vi "Test--wink.vi"() -> ()   [LabVIEW 2024, in "Flexi-Flow Modbus TCP API.lvlib"]
uses:
  Flexi-Flow Modbus TCP API.lvlib
  ca-ec-test-stand/Dependencies/gmodbustcp-main/Sources/Lvlib/ModBusVIEWoTCP.lvlib
panel:
  out "Word":i16
  out "Information out":T1 {"Unit identifier" max=247; "exceptionCode" max=247}
  in  "Word address":u16 format="%x"
  in  "Word (0)":i16
  in  "Network":T2={"server address"="192.168.100.10", "remote port (502)"=502}
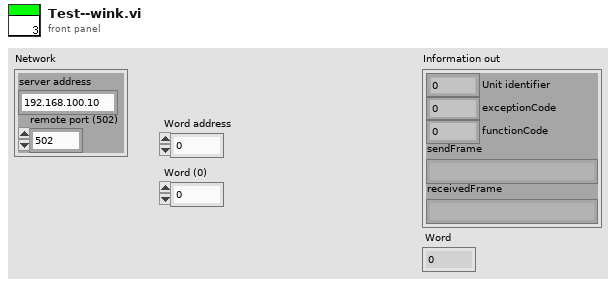
[diagram p1: front panel]
types:
  T1 = cluster{"Unit identifier":u8, "exceptionCode":u8, "functionCode":u8, "sendFrame":string, "receivedFrame":string}
  T2 = cluster{"server address":string, "remote port (502)":u16}
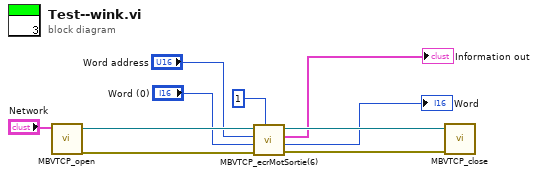
[diagram p0: block diagram]
diagram:
  n1 = call "MBVTCP_open.vi"("Network"="Network") -> ("error out"=w6:errorcluster, "NetRefTCP out"=w9:refnum<k5>)  [unwired: 2 in, 7 out]
  n2 = call "MBVTCP_ecrMotSortie(6).vi"("Unit identifier (x1)"=u8 1, "error in"=w6, "Word (0)"="Word (0)", "Word address"="Word address", "NetRefTCP in"=w9) -> ("error out"=w7:errorcluster, "Word"=→"Word":i16, "Information out"=→"Information out":T1, "NetRefTCP out"=w8:refnum<k5>)  [unwired: 1 in, 2 out]
  n3 = call "MBVTCP_close.vi"("error in"=w7, "NetRefTCP in"=w8) -> ()  [unwired: 10 out]
